vi "enqueue_dp_data.vi"(0 "dP Queue":refnum<queue>, 1 "dP Recording Progress":refnum<vi>, 2 "MeasurementData":dbl[][](array[numeric]), 3 "# of Samples":dbl format="%#_13g", 4 "Record dP Data":refnum<vi>) -> ()   [LabVIEW 2017]
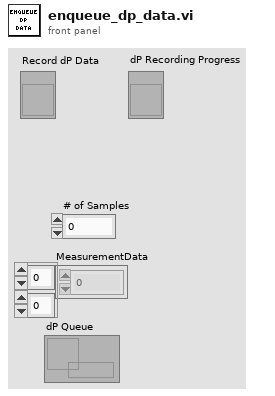
[diagram p1: front panel]
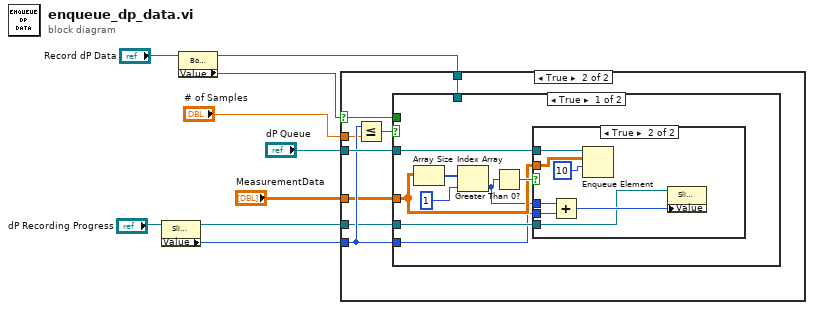
[diagram p0: block diagram]
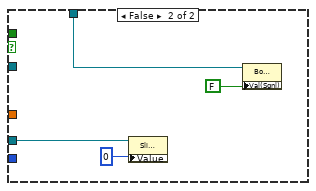
[diagram p4: hidden frame]
diagram:
  n1 = property class="Slide (strict)"(reference="dP Recording Progress") -> (reference out=w2:refnum<vi>, "Value"=w3:u32)  [unwired: 1 in, 1 out]
  n2 = property class="Bool (strict)"(reference="Record dP Data") -> (reference out=w1:refnum<vi>, "Value"=w5:bool)  [unwired: 1 in, 1 out]
  n3 = case shown="True" w5 {
    selector: w5 -> [_ w12]
    tunnel: "dP Queue" -> [_ w17]
    tunnel: w3 -> [_ w16]
    tunnel: "MeasurementData" -> [_ w15]
    tunnel: "# of Samples" -> [_ w13]
    tunnel: w2 -> [_ w11]
    tunnel: w1 -> [_ w10]
    frame False {
    }
    frame True {
      n4 = Less Or Equal?(x=w16, y=w13) -> (x <= y?=w14:bool)
      n5 = case shown="True" w14 {
        tunnel: w17 -> [w25 _]
        tunnel: w16 -> [w21 _]
        tunnel: w15 -> [w23 _]
        tunnel: w12 -> [_ _]
        tunnel: w11 -> [w22 w36]
        tunnel: w10 -> [_ w33]
        frame True {
          n6 = Array Size(array=w23) -> (size(s)=w20:i32[])
          n7 = Index Array(array=w20, index=1) -> (element=w18:i32)
          n8 = Greater Than 0?(x=w18) -> (x > 0?=w24:bool)
          n9 = case shown="True" w24 {
            tunnel: w25 -> [_ w31]
            tunnel: w21 -> [_ w30]
            tunnel: w23 -> [_ w29]
            tunnel: w22 -> [_ w27]
            tunnel: w18 -> [_ w26]
            frame False {
            }
            frame True {
              n10 = Add(x=w26, y=w30) -> (x+y=w28:u32)
              n11 = Enqueue Element(queue=w31, element=w29, timeout in ms (-1)=10) -> ()  [unwired: 1 in, 3 out]
              n12 = property class="Slide (strict)"(reference=w27, "Value"=w28) -> ()  [unwired: 1 in, 2 out]
            }
          }
        }
        frame False {
          n13 = property class="Slide (strict)"(reference=w36, "Value"=u32 0 ("dP Recording Progress")) -> ()  [unwired: 1 in, 2 out]
          n14 = property class="Bool (strict)"(reference=w33, "Val(Sgnl)"=FALSE ("Value (Signaling)")) -> ()  [unwired: 1 in, 2 out]
        }
      }
    }
  }
